vi "USBMotorController.vi"(8 "error in":errorcluster, 11 "MotorAddress":i32) -> (0 "error out":errorcluster)   [LabVIEW 2013]
uses:
  <instrlib>/arcus/ArcusUsbComm.llb/commands.ctl
panel:
  in  "Enum":T1(ring)
  in  "Parameter":i32
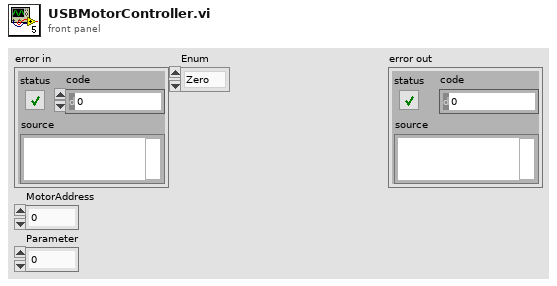
[diagram p1: front panel]
types:
  T1 = enum16{"Zero", "MoveTo", "Halt", "ClearError", "PowerUp", "Select"}
  T2 = typedef "commands.ctl" = enum16{"clear error", "constant jog(-)", "constant jog(+)", "get acceleration", "get actual current", "get device id", "get digital input status", "get digial inputs status", "get dig output status", "get digital outputs status", "get firmware ver", "get high speed", "get idle current", "get low speed", "get micro step", "get motor status", "get move mode", "get polarity", "get position", "get product id", "get power status", "get run current", "get status", "home(-)", "home(+)", "move to position", "power down", "power up", "set acceleration", "set device id", "set digital output", "set digital outputs", "set high speed", "set idle current", "set low speed", "set move mode absolute", "set move mode increment", "set polarity", "set position", "set run current", "stop immediate", "stop slow", "store to memory"}
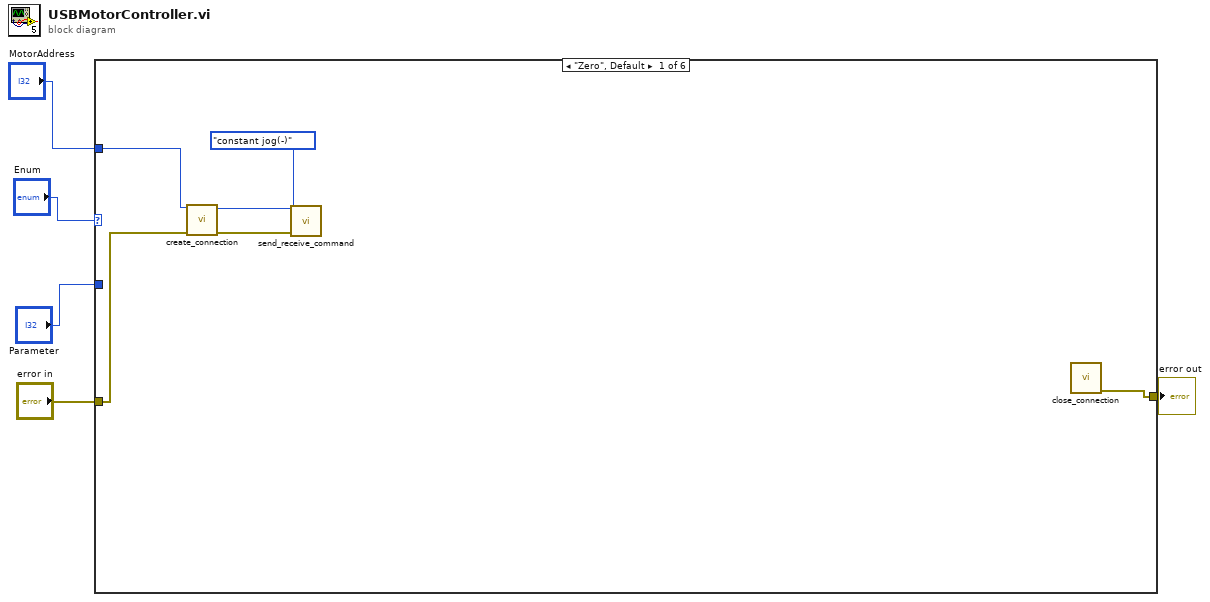
[diagram p0: block diagram]
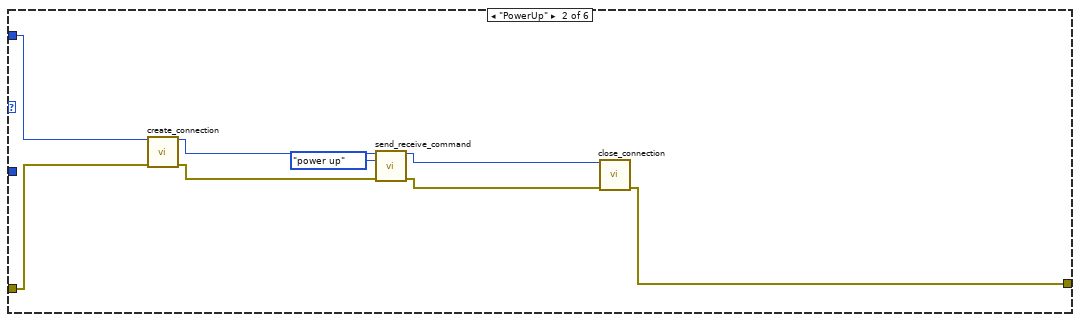
[diagram p2: hidden frame]
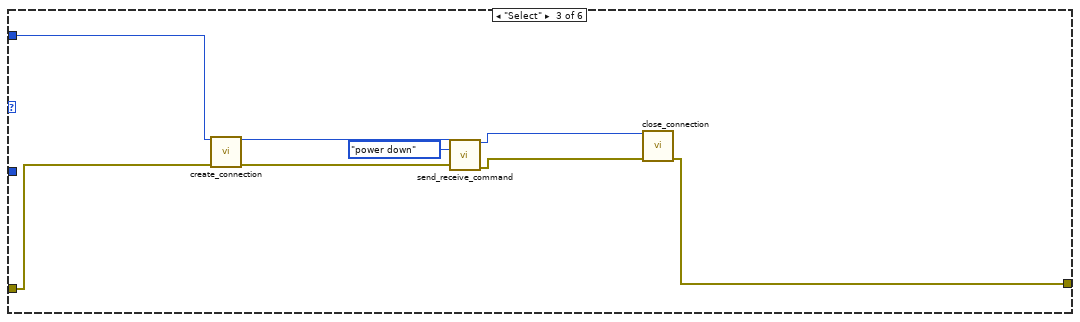
[diagram p3: hidden frame]
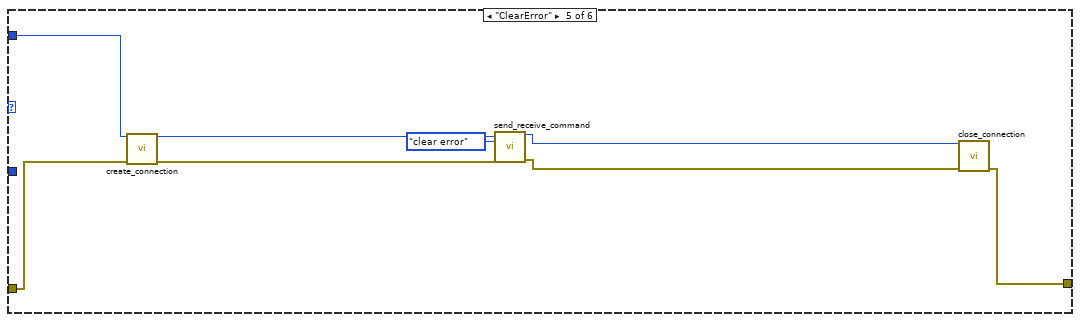
[diagram p5: hidden frame]
diagram:
  n1 = case shown="\"Zero\", Default" "Enum" {
    tunnel: "error in" -> [w10 w16 w24 _ w34 _]
    tunnel: [w11 w12 w20 _ w31 _] -> w4
    tunnel: "MotorAddress" -> [w9 w19 w25 _ w35 _]
    tunnel: "Parameter" -> [_ _ _ _ _ _]
    frame "Zero", Default {
      n2 = call <instrlib>:"create_connection.vi"("device_index (def=0)"=w9, "error in (no error)"=w10) -> ("reference"=w7:i32, "error out"=w8:errorcluster)  [unwired: 12 in]
      n3 = call <instrlib>:"send_receive_command.vi"("reference (in)"=w7, "command"=commands."constant jog(-)", "error in (no error)"=w8) -> ()  [unwired: 8 in, 5 out]
      n4 = call <instrlib>:"close_connection.vi"() -> ("error out"=w11:errorcluster)  [unwired: 15 in]
    }
    frame "PowerUp" {
      n5 = call <instrlib>:"create_connection.vi"("device_index (def=0)"=w19, "error in (no error)"=w16) -> ("reference"=w18:i32, "error out"=w15:errorcluster)  [unwired: 12 in]
      n6 = call <instrlib>:"send_receive_command.vi"("reference (in)"=w18, "command"=commands."power up", "error in (no error)"=w15) -> ("reference (dup)"=w17:i32, "error out"=w14:errorcluster)  [unwired: 8 in, 3 out]
      n7 = call <instrlib>:"close_connection.vi"("reference"=w17, "error in (no error)"=w14) -> ("error out"=w12:errorcluster)  [unwired: 13 in]
    }
    frame "Select" {
      n8 = call <instrlib>:"create_connection.vi"("device_index (def=0)"=w25, "error in (no error)"=w24) -> ("reference"=w27:i32, "error out"=w23:errorcluster)  [unwired: 12 in]
      n9 = call <instrlib>:"send_receive_command.vi"("reference (in)"=w27, "command"=commands."power down", "error in (no error)"=w23) -> ("reference (dup)"=w26:i32, "error out"=w22:errorcluster)  [unwired: 8 in, 3 out]
      n10 = call <instrlib>:"close_connection.vi"("reference"=w26, "error in (no error)"=w22) -> ("error out"=w20:errorcluster)  [unwired: 13 in]
    }
    frame "Halt" {
    }
    frame "ClearError" {
      n11 = call <instrlib>:"create_connection.vi"("device_index (def=0)"=w35, "error in (no error)"=w34) -> ("reference"=w33:i32, "error out"=w30:errorcluster)  [unwired: 12 in]
      n12 = call <instrlib>:"send_receive_command.vi"("reference (in)"=w33, "command"=commands."clear error", "error in (no error)"=w30) -> ("reference (dup)"=w32:i32, "error out"=w29:errorcluster)  [unwired: 8 in, 3 out]
      n13 = call <instrlib>:"close_connection.vi"("reference"=w32, "error in (no error)"=w29) -> ("error out"=w31:errorcluster)  [unwired: 13 in]
    }
    frame "MoveTo" {
    }
  }
  "error out" <- w4
